vi "RTS Sys Time ON.vi"(8 "Error In":errorcluster, 10 "length":i32=4, 11 "Point File in":T1[](array[typedef])) -> (0 "Error Out":errorcluster, 3 "Point File out":T1[](array[typedef]))   [LabVIEW 2019]
uses:
  Type Definitions/RTS Point File.ctl
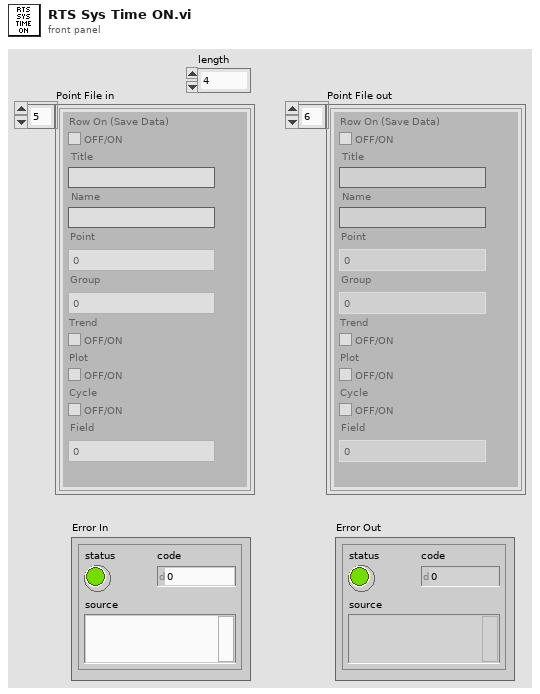
[diagram p1: front panel]
types:
  T1 = typedef "RTS Point File.ctl" = cluster{"Title":string, "Name":string, "Point":u8, "Plot":bool, "Trend":bool, "Cycle":bool, "Field":u8, "Row On (Save Data)":bool, "Group":u8}
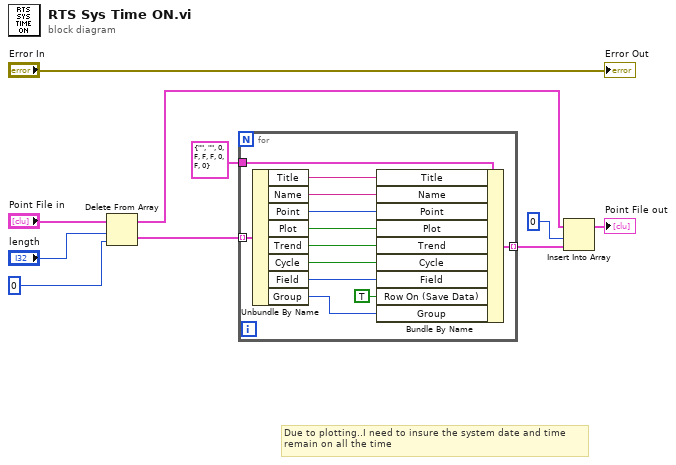
[diagram p0: block diagram]
diagram:
  # "Due to plotting..I need to insure the system date and time\nremain on all the time"
  n1 = Delete From Array(array="Point File in", length="length", index=0) -> (deleted portion=w6:T1[], array with subset deleted=w7:T1[])
  n2 = for {
    tunnel: T1 {"Title"="", "Name"="", "Point"=0, "Plot"=FALSE, "Trend"=FALSE, "Cycle"=FALSE, "Field"=0, "Row On (Save Data)"=FALSE, "Group"=0} ("Point File Input 2") -> [w22]
    tunnel: w6 -> [w21] mode=indexing
    tunnel: [w11] -> w9 mode=indexing
    n3 = Unbundle By Name(w21) -> ("Title"=w20:string, "Name"=w19:string, "Point"=w18:u8, "Plot"=w17:bool, "Trend"=w16:bool, "Cycle"=w15:bool, "Field"=w14:u8, "Group"=w12:u8)
    n4 = Bundle By Name(cluster=w22, "Title"=w20, "Name"=w19, "Point"=w18, "Plot"=w17, "Trend"=w16, "Cycle"=w15, "Field"=w14, "Row On (Save Data)"=TRUE, "Group"=w12) -> (w11:T1)
  }
  n5 = Insert Into Array(array=w7, index=0, new element=w9) -> (→"Point File out":T1[])
  "Error Out" <- "Error In"
